vi "Log Data.vi"(8 "error in (no error)":errorcluster, 10 "Data Queue":refnum<queue>, 11 "Logging Configuration":T1) -> (0 "error out":errorcluster, 3 "Logging Configuration 2":T1)   [LabVIEW 2018, in "System Logging.lvlib" / "Logging.lvlib"]
doc: "This VI uses the TDMS Write function to write data to a TDMS file."
uses:
  Logging.lvlib
  Logging Configuration.ctl
  <vilib>/Waveform/WDTOps.llb/WDT Get Waveform Time Array DBL.vi
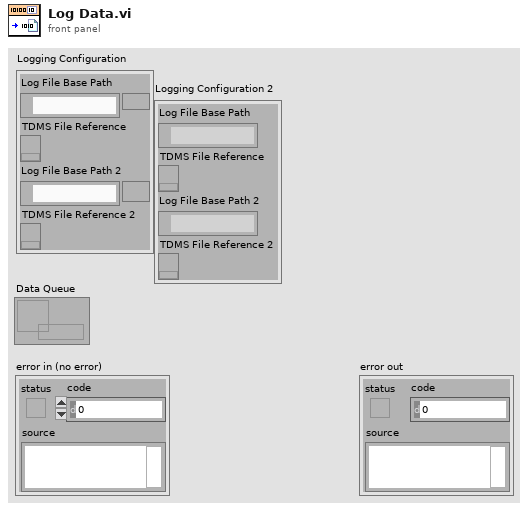
[diagram p1: front panel]
types:
  T1 = typedef "System Logging.lvlib/Logging.lvlib/Logging Configuration.ctl" = cluster{"Log File Base Path":path, "TDMS File Reference":refnum<k34>, "Log File Base Path 2":path, "TDMS File Reference 2":refnum<k34>}
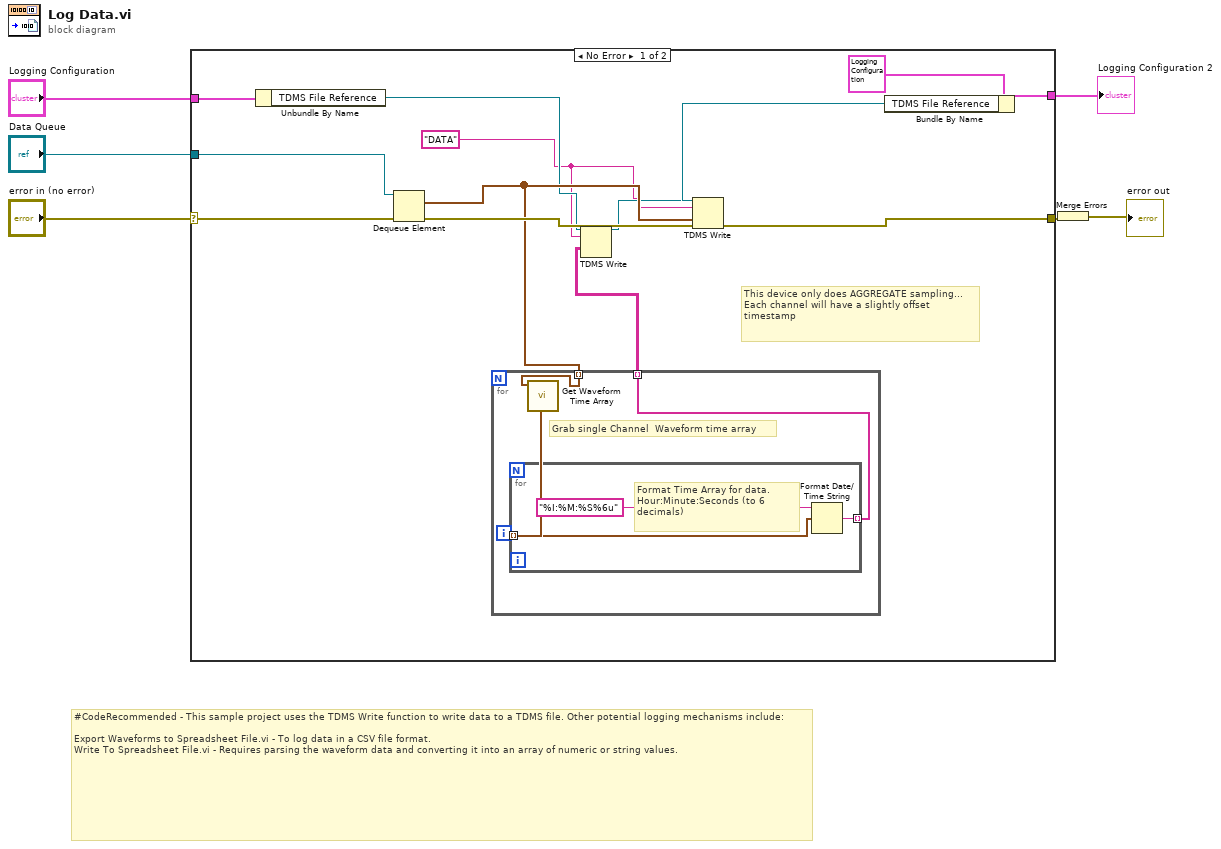
[diagram p0: block diagram]
diagram:
  # "#CodeRecommended - This sample project uses the TDMS Write function to write data to a TDMS file. Other potential logging mechanisms include:\n\nExport Waveforms to Spreadsheet File.vi - To log data in a CSV file format.\nWrite To Spreadsheet File.vi - Requires parsing the waveform data and converting it into an array of numeric or string values."
  n1 = case shown="No Error" "error in (no error)" {
    selector: "error in (no error)" -> [w18 w27]
    tunnel: "Logging Configuration" -> [w19 w26]
    tunnel: "Data Queue" -> [w17 _]
    tunnel: [w16 w27] -> w3
    tunnel: [w14 w26] -> w1
    frame No Error {
      w8 = "DATA"
      # "This device only does AGGREGATE sampling... Each channel will have a slightly offset timestamp"
      n2 = Unbundle By Name(w19) -> ("TDMS File Reference"=w10:refnum<k34>)
      n3 = Dequeue Element(queue=w17, error in (no error)=w18) -> (element=w11:waveform(dbl)[], error out=w12:errorcluster)  [unwired: 1 in, 2 out]
      n4 = for {
        tunnel: w11 -> [w22] mode=indexing
        tunnel: [w20] -> w7 mode=indexing
        # "Grab single Channel  Waveform time array"
        n5 = call-poly <vilib>:"Get Waveform Time Array.vi"("waveform in"=w22) -> ("X array"=w21:timestamp[])  [unwired: 9 in, 1 out]
        n6 = for {
          tunnel: w21 -> [w25] mode=indexing
          tunnel: [w24] -> w20 mode=indexing
          # "Format Time Array for data. Hour:Minute:Seconds (to 6 decimals)"
          n7 = Format Date/Time String(time format string (%c)="%I:%M:%S%6u", seconds (now)=w25) -> (date/time string=w24:string)  [unwired: 1 in]
        }
      }
      n8 = TDMS Write(0:w10, 5:w8, 9:w7) -> (4:w9:refnum<k34>)  [unwired: 3 in, 3 out]
      n9 = TDMS Write(0:w9, 5:w8, 9:w11, 11:w12) -> (4:w15:refnum<k34>, 15:w16:errorcluster)  [unwired: 2 in, 2 out]
      n10 = Bundle By Name(cluster=T1 {"Log File Base Path"=path "", "TDMS File Reference"=refnum, "Log File Base Path 2"=path "C:/Users/J.Schwartz/Documents/LabVIEW Data/Space Station Test/Test Data/Test 1_2017_06_13_16_01_42.tdms", "TDMS File Reference 2"=refnum} ("Logging Configuration"), "TDMS File Reference"=w15) -> (w14:T1)
    }
    frame Error {
    }
  }
  "Logging Configuration 2" <- w1
  n11 = Merge Errors(w3) -> (→"error out":errorcluster)
